vi "Query Error.vi"(8 "error in (no error)":errorcluster, 11 "3446X in":refnum<class "3446X.lvclass">) -> (0 "error out":errorcluster, 1 "Error Message":string, 2 "Error Code":i32, 3 "3446X out":refnum<class "3446X.lvclass">)   [LabVIEW 2018, in "3446X.lvlib" / "3446X.lvclass"]
uses:
  3446X.lvclass
  3446X.lvclass/3446X.ctl
  <instrlib>/Agilent 3446X Series/Agilent 3446X Series.lvlib
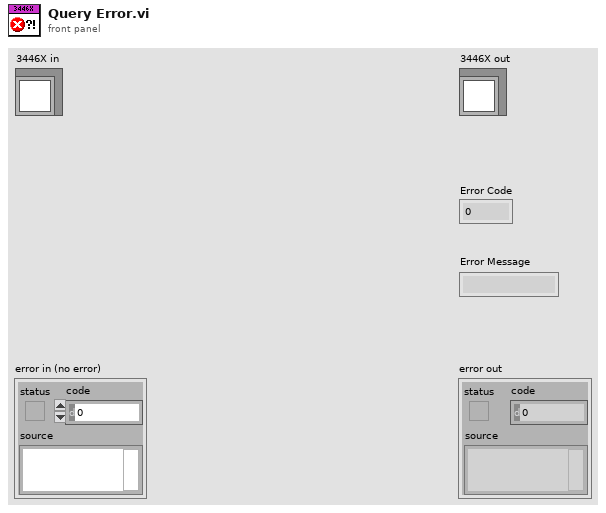
[diagram p1: front panel]
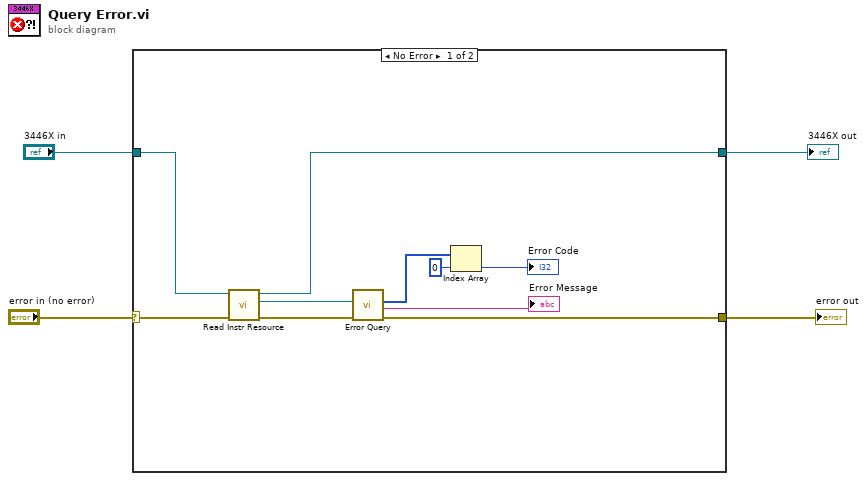
[diagram p0: block diagram]
diagram:
  n1 = case shown="No Error" "error in (no error)" {
    selector: "error in (no error)" -> [w14 w16]
    tunnel: [w6 w16] -> w3
    tunnel: [w5 w15] -> w2
    tunnel: "3446X in" -> [w13 w15]
    frame No Error {
      n2 = call "Read Instr Resource.vi"("error in (no error)"=w14, "3446X in"=w13) -> ("error out"=w11:errorcluster, "Instr Resource"=w12:refnum<visa-resource-name>, "3446X out"=w5:refnum<class "3446X.lvclass">)  [unwired: 7 in]
      n3 = call <instrlib>:"Error Query.vi"("error in (no error)"=w11, "VISA resource name"=w12) -> ("error out"=w6:errorcluster, "Error Message"=→"Error Message":string, "Error Code"=w10:i32[])  [unwired: 6 in, 1 out]
      n4 = Index Array(array=w10, index=0) -> (element=→"Error Code":i32)
    }
    frame Error {
    }
  }
  "error out" <- w3
  "3446X out" <- w2
